vi "Untitled 6.vi"() -> ()   [LabVIEW 2021]
uses:
  Drivers/Arduino_Pulse_Generator/Configurate/Register_1.ctl
  Drivers/Arduino_Pulse_Generator/Configurate/Register_2.ctl
  Drivers/Arduino_Pulse_Generator/Configurate/Channel_Pulse_Stream.ctl
  Main/Ver_1/Config_File_Paths.ctl
  <instrlib>/Zurich Instruments LabOne/Public/Modules/ziModGetDoubleData.vi
  <instrlib>/Zurich Instruments LabOne/Public/Utility/ziTicksToS_vector.vi
  <instrlib>/Zurich Instruments LabOne/Zurich Instruments LabOne.lvlib
panel:
  out "progress":dbl(slide) scale=0.0..1.0
  out "XY Graph":cluster{"Timestamp(s)":dbl[], "Value":dbl[]}(graph)
  out "error out":errorcluster
  in  "Config files paths":T1={"ZI config file (.ini)"="Config_Ver_1\\Zurich_params.ini", "Keithley config file (.ini)"="Config_Ver_1\\Keithley_params.ini", "Arduino config file (.ini)"="Config_Ver_1\\pulse_sequence.ini"}
  in  "Resource Address":T2={"ZI Address"="DEV714", "VISA Keithley"="KEITHLEY", "VISA Arduino PG"="Arduino_PGen"}
  in  "error in":errorcluster
  out "Pulse sequence indicator":T3[](array[typedef]) {"channel" min=2 max=13 step=1}
  in  "Time unit":string(combo)="ms"
  out "Init States":T6
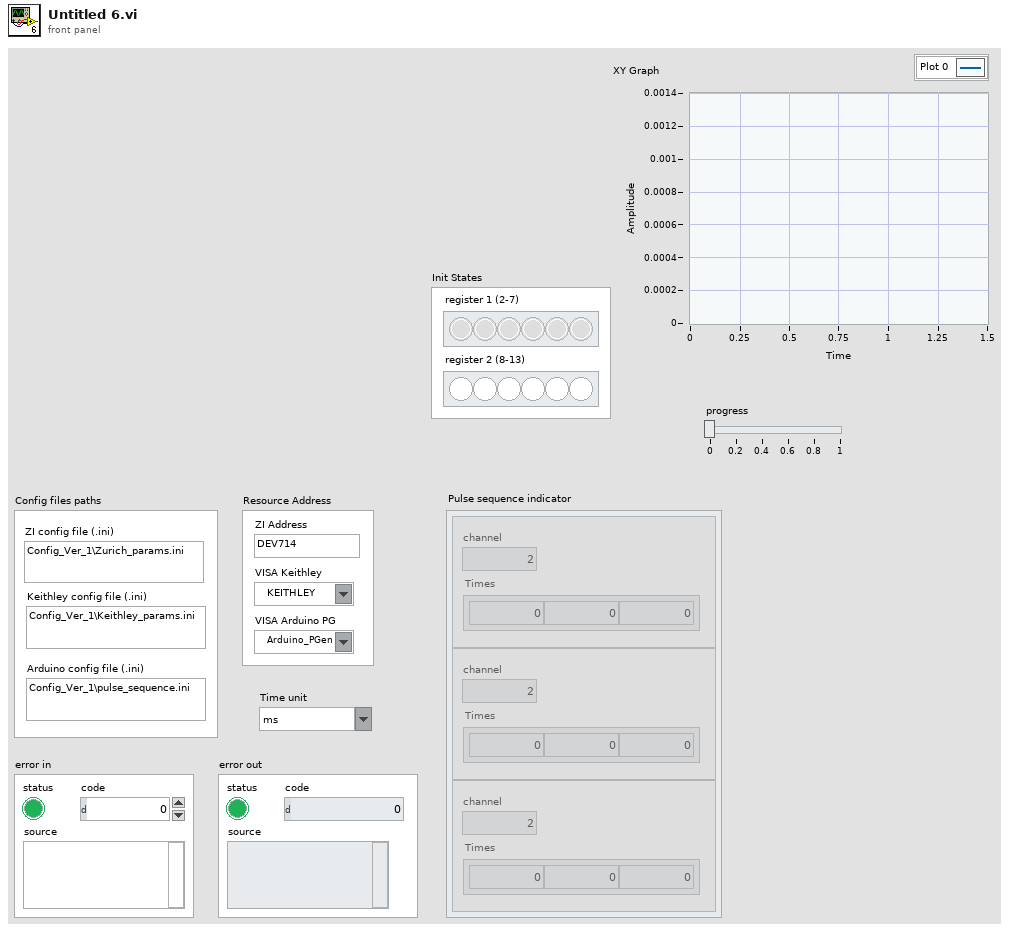
[diagram p1: front panel]
types:
  T1 = typedef "Config_File_Paths.ctl" = cluster{"ZI config file (.ini)":string, "Keithley config file (.ini)":string, "Arduino config file (.ini)":string}
  T2 = cluster{"ZI Address":string, "VISA Keithley":refnum<visa-resource-name>, "VISA Arduino PG":refnum<visa-resource-name>}
  T3 = typedef "Channel_Pulse_Stream.ctl" = cluster{"Times":dbl[], "channel":u8}
  T4 = typedef "Register_1.ctl" = bool[]
  T5 = typedef "Register_2.ctl" = bool[]
  T6 = cluster{"register 1 (2-7)":T4, "register 2 (8-13)":T5}
  T7 = typedef "Resources.ctl" = cluster{"ZI Handle":T8, "ZI ModHandle":T9, "VISA arduino":refnum<visa-resource-name>, "VISA Keithley":refnum<visa-resource-name>}
  T8 = typedef "Zurich Instruments LabOne.lvlib/ziTypeHandle.ctl" = cluster{"handleValid":bool, "Conn":u64, "Path Prefix":string, "Handle":u64, "Connected":bool, "Clockbase(s)":dbl}
  T9 = typedef "Zurich Instruments LabOne.lvlib/ziTypeModHandle.ctl" = cluster{"handleValid":bool, "Conn":u64, "ModHandle":u64, "moduleID":string, "Path Prefix":string}
  T10 = typedef "Zurich Instruments LabOne.lvlib/ziTypeModResults.ctl" = cluster{"PathArray":string[], "ValueType":T11, "NoOfResults":u64, "ziGenericHeader":T12[]}
  T11 = typedef "Zurich Instruments LabOne.lvlib/ziTypePollType.ctl" = enum16{"NONE", "DOUBLE_DATA", "INTEGER_DATA", "DEMOD_SAMPLE", "SCOPE_WAVE_HF2", "AUXIN_SAMPLE", "DIO_SAMPLE", "BYTE_ARRAY", "PWA_WAVE", "9", "10", "11", "12", "13", "14", "15", "TREE_CHANGE_DEPRI", "17", "ERROR", "19", "20", "21", "22", "23", "24", "25", "26", "27", "28", "29", "30", "31", "DOUBLE_DATA_TS", "INTEGER_DATA_TS", "34", "SCOPE_WAVE", "SCOPE_WAVE_EX", "37", "BYTE_ARRAY_TS", "39", "40", "41", "42", "43", "44", "45", "CNT_DATA", "47", "TREE_CHANGE", "49", "50", "51", "52", "53", "54", "55", "56", "57", "58", "59", "60", "61", "62", "63", "SWEEPER_DATA", "SPECTRUM_DATA", "ADVISOR_DATA", "VECTOR_DATA", "IMP_DATA"}
  T12 = typedef "Zurich Instruments LabOne.lvlib/ziTypeModGenericHeader.ctl" = cluster{"HeaderType":enum8{"HEADER_TYPE_NONE", "HEADER_TYPE_SWTRIGGER", "HEADER_TYPE_SWEEPER"}, "SampleFormat":u8, "SystemTime":timestamp, "CreatedTimeStamp":u64, "ChangedTimeStamp":u64, "Flags":u32, "ChunkSizeBytes":u64, "Name":string, "Status":u32, "GroupIndex":u32, "Color":u32, "ActiveRow":u32, "TriggerNumber":u64, "GridRows":u32, "GridCols":u32, "GridMode":u32, "GridOperation":u32, "GridDirection":u32, "GridRepetitions":u32, "GridColDelta":dbl, "GridColOffset":dbl, "GridRowDelta":dbl, "GridRowOffset":dbl, "Bandwidth":dbl, "Center":dbl, "Nenbw":dbl}
  T13 = typedef "Zurich Instruments LabOne.lvlib/ziTypeDoubleDataTS.ctl" = cluster{"Timestamp (ticks)":u64[], "Value":dbl[]}
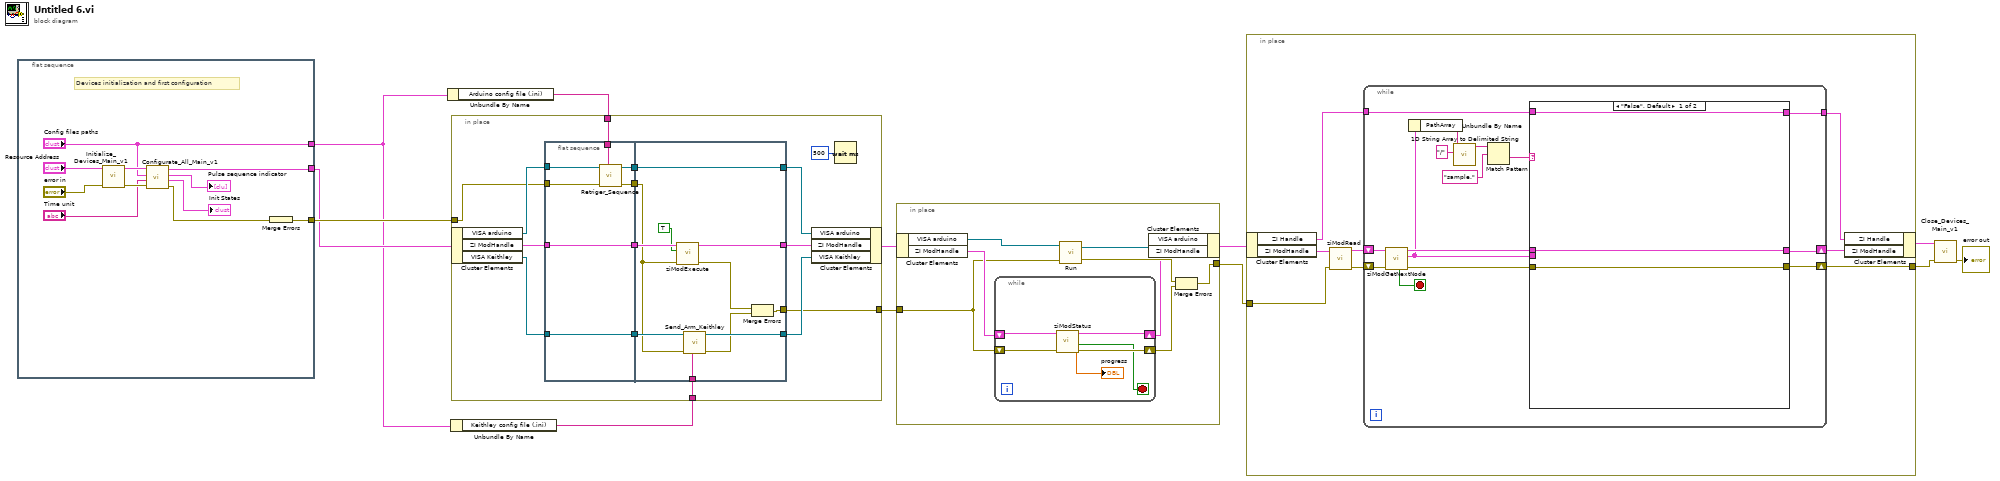
[diagram p0: block diagram]
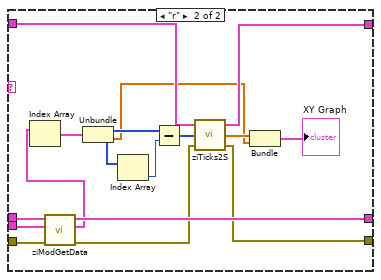
[diagram p2: hidden frame]
diagram:
  n1 = flat-sequence {
    tunnel: [w17] -> w10
    tunnel: [w15] -> w11
    tunnel: ["Config files paths"] -> w8
    frame #0 {
      # "Devices initialization and first configuration"
      n2 = call "Initialize_Devices_Main_v1.vi"("error in"="error in", "Resource Address"="Resource Address") -> ("error out"=w20:errorcluster, "Resources"=w21:T7)  [unwired: 8 in]
      n3 = call "Configurate_All_Main_v1.vi"("error in"=w20, "Time unit"="Time unit", "Config files paths"="Config files paths", "Resources in"=w21) -> ("error out"=w16:errorcluster, "Init States"=→"Init States":T6, "Pulse sequence"=→"Pulse sequence indicator":T3[], "Resources out"=w17:T7)  [unwired: 4 in]
      n4 = Merge Errors(w16) -> (w15:errorcluster)
    }
  }
  n5 = Unbundle By Name(w8) -> ("Arduino config file (.ini)"=w9:string)
  n6 = Unbundle By Name(w8) -> ("Keithley config file (.ini)"=w7:string)
  n7 = in-place {
    in-place-border: w11 -> [w37]
    in-place-border: [w33] -> w5
    in-place-border: w9 -> [w32]
    in-place-border: w7 -> [w24]
    n8 = in-place-cluster #1(w10) -> ("VISA arduino"=w38:refnum<visa-resource-name>, "ZI ModHandle"=w31:T9, "VISA Keithley"=w28:refnum<visa-resource-name>)
    n9 = flat-sequence {
      tunnel: w38 -> [w41]
      tunnel: w37 -> [w40]
      tunnel: [w39] -> w36
      tunnel: w32 -> [w43]
      tunnel: w31 -> [w45]
      tunnel: [w45] -> w30
      tunnel: w28 -> [w44]
      tunnel: [w44] -> w29
      tunnel: [w42] -> w26
      tunnel: w36 -> [w47]
      tunnel: [w49] -> w34
      tunnel: [w55] -> w35
      tunnel: [w54] -> w33
      tunnel: w30 -> [w53]
      tunnel: w29 -> [w50]
      tunnel: [w51] -> w27
      tunnel: w26 -> [w51]
      tunnel: w24 -> [w48]
      frame #0 {
        n10 = call "Retriger_Sequence.vi"("Filename (.ini)"=w43, "error in"=w40, "VISA arduino in"=w41) -> ("error out"=w39:errorcluster, "VISA arduino out"=w42:refnum<visa-resource-name>)  [unwired: 4 in, 3 out]
      }
      frame #1 {
        n11 = call <instrlib>:"ziModExecute.vi"("Error In"=w47, "Modal (F)"=TRUE, "ziModHandle In"=w53) -> ("Error Out"=w56:errorcluster, "ziModHandle Out"=w55:T9)  [unwired: 6 in]
        n12 = call "Send_Arm_Keithley.vi"("Filename (.ini)"=w48, "error in"=w47, "Keithley VISA in"=w50) -> ("error out"=w46:errorcluster, "Keithley VISA out"=w49:refnum<visa-resource-name>)  [unwired: 6 in, 1 out]
        n13 = Merge Errors(w56, w46) -> (w54:errorcluster)
      }
    }
    n14 = in-place-cluster #1("VISA arduino"=w27, "ZI ModHandle"=w35, "VISA Keithley"=w34) -> (w6:T7)
    n15 = Wait (ms)(milliseconds to wait=u32 500) -> ()  [unwired: 1 out]
  }
  n16 = in-place {
    in-place-border: w5 -> [w61]
    in-place-border: [w58] -> w3
    n17 = in-place-cluster #2(w6) -> ("VISA arduino"=w64:refnum<visa-resource-name>, "ZI ModHandle"=w62:T9)
    n18 = while {
      shift-right: [w69] -> w57
      shift-left: w62 -> [w70]
      shift-right: [w67] -> w59
      shift-left: w61 -> [w68]
      stop <- w65 stop-if-true
      n19 = call <instrlib>:"ziModStatus.vi"("Error In"=w68, "ModHandle IN"=w70) -> ("Error Out"=w67:errorcluster, "Finished?"=w65:bool, "Progress (unity)"=→"progress":dbl, "ModHandle Out"=w69:T9)  [unwired: 5 in]
    }
    n20 = call "Run.vi"("error in"=w61, "VISA arduino in"=w64) -> ("error out"=w60:errorcluster, "VISA arduino out"=w63:refnum<visa-resource-name>)  [unwired: 1 in]
    n21 = in-place-cluster #2("VISA arduino"=w63, "ZI ModHandle"=w57) -> (w4:T7)
    n22 = Merge Errors(w60, w59) -> (w58:errorcluster)
  }
  n23 = in-place {
    in-place-border: w3 -> [w77]
    in-place-border: [w71] -> w1
    n24 = in-place-cluster #3(w4) -> ("ZI Handle"=w74:T8, "ZI ModHandle"=w78:T9)
    n25 = call <instrlib>:"ziModRead.vi"("error in"=w77, "ziModHandle In"=w78) -> ("error out"=w76:errorcluster, "ziModHandle Out"=w75:T9)  [unwired: 8 in]
    n26 = while {
      shift-right: [w82] -> w72
      shift-left: w75 -> [w89]
      shift-right: [w79] -> w71
      shift-left: w76 -> [w88]
      tunnel: w74 -> [w81]
      tunnel: [w80] -> w73
      stop <- w83 stop-if-true
      n27 = call <instrlib>:"ziModGetNextNode.vi"("Error In"=w88, "ModHandle In"=w89) -> ("Error Out"=w84:errorcluster, "ModResults"=w85:T10, "ModHandle Out"=w86:T9, "NoData"=w83:bool)  [unwired: 6 in]
      n28 = Unbundle By Name(w85) -> ("PathArray"=w92:string[])
      n29 = call <vilib>:"1D String Array to Delimited String.vi"("delimiter"="/", "string array"=w92) -> ("delimited string"=w93:string)  [unwired: 9 in]
      n30 = Match Pattern(string=w93, regular expression="sample.") -> (after substring=w87:string)  [unwired: 1 in, 3 out]
      n31 = case shown="\"False\", Default" w87 {
        tunnel: w86 -> [w95 w112]
        tunnel: w85 -> [_ w111]
        tunnel: w84 -> [w94 w110]
        tunnel: [w95 w109] -> w82
        tunnel: w81 -> [w96 w108]
        tunnel: [w96 w107] -> w80
        tunnel: [w94 w100] -> w79
        frame "False", Default {
        }
        frame "r" {
          n32 = call-poly <instrlib>:"ziModGetData.vi"("Error In"=w110, "ModResults"=w111, "ModHandle In"=w112) -> ("Error Out"=w101:errorcluster, "DoubleSample"=w106:T13[], "ModHandle Out"=w109:T9)  [unwired: 4 in, 2 out]
          n33 = Index Array(array=w106) -> (element=w105:T13)  [unwired: 1 in]
          n34 = Unbundle(w105) -> ("Timestamp (ticks)"=w102:u64[], "Value"=w98:dbl[])
          n35 = Index Array(array=w102) -> (element=w103:u64)  [unwired: 1 in]
          n36 = Subtract(x=w102, y=w103) -> (x-y=w104:u64[])
          n37 = call-poly <instrlib>:"ziTicks2S.vi"("Error In"=w101, "Timestamp (ticks)"=w104, "Handle In"=w108) -> ("Error Out"=w100:errorcluster, "Timestamp(s)"=w99:dbl[], "Handle Out"=w107:T8)
          n38 = Bundle("Timestamp(s)"=w99, "Value"=w98) -> (→"XY Graph":cluster{"Timestamp(s)":dbl[], "Value":dbl[]})  [unwired: 1 in]
        }
      }
    }
    n39 = in-place-cluster #3("ZI Handle"=w73, "ZI ModHandle"=w72) -> (w2:T7)
  }
  n40 = call "Close_Devices_Main_v1.vi"("error in"=w1, "Resources in"=w2) -> ("error out"=→"error out":errorcluster)  [unwired: 9 in]
